vi "Timer.vi"() -> ()   [LabVIEW 2012]
uses:
  SAPI_TTS_Library_v110/SAPI TTS Library/SubVIs/SAPI_Speak_Text_String_SubVI.vi
  <vilib>/Instr/_visa.llb/VISA Configure Serial Port (Instr).vi
  SAPI_TTS_Library_v110/SAPI TTS Library/SAPI.TTS.lvlib
panel:
  in  "Boolean 2":bool
  out "Start":bool
  out "Speaking... 3":bool
  in  "Volume 3":i32(slide)=100 min=0 max=100 scale=0.0..100.0
  in  "Rate 3":i32(slide) min=-10 max=10 scale=-10.0..10.0
  in  "Output Device 3":u16(ring) items=["Speakers (Realtek High Definition Audio)"]
  in  "TTS Voice 3":u16(ring) items=["Microsoft Anna - English (United States)"]
  out "Speaking... 2":bool
  in  "Volume 2":i32(slide)=100 min=0 max=100 scale=0.0..100.0
  in  "Rate 2":i32(slide) min=-10 max=10 scale=-10.0..10.0
  in  "Output Device 2":u16(ring) items=["Speakers (Realtek High Definition Audio)"]
  in  "TTS Voice 2":u16(ring) items=["Microsoft Anna - English (United States)"]
  in  "String to Speak 2":string
  in  "Boolean":bool
  out "最高纪录 (Max Record)":dbl format="%.6f"
  in  "String to Speak":string
  in  "TTS Voice":u16(ring) items=["Microsoft Anna - English (United States)"]
  in  "Output Device":u16(ring) items=["Speakers (Realtek High Definition Audio)"]
  in  "Rate":i32(slide) min=-10 max=10 scale=-10.0..10.0
  in  "Volume":i32(slide)=100 min=0 max=100 scale=0.0..100.0
  out "Speaking...":bool
  out "已用时间 (Elasped Time)":dbl format="%.3f"
  out "LastTimeDetected":dbl
  out "单圈时间 (Lap Time)":dbl format="%.3f"
  in  "启动 / 停止":bool
  in  "赛道总长度":dbl
  in  "串口号":refnum<visa-resource-name>
  out "平均速度 (Average Speed)":dbl format="%.6f"
  # "武汉工程大学 \n”Freescale“赛道计时器"
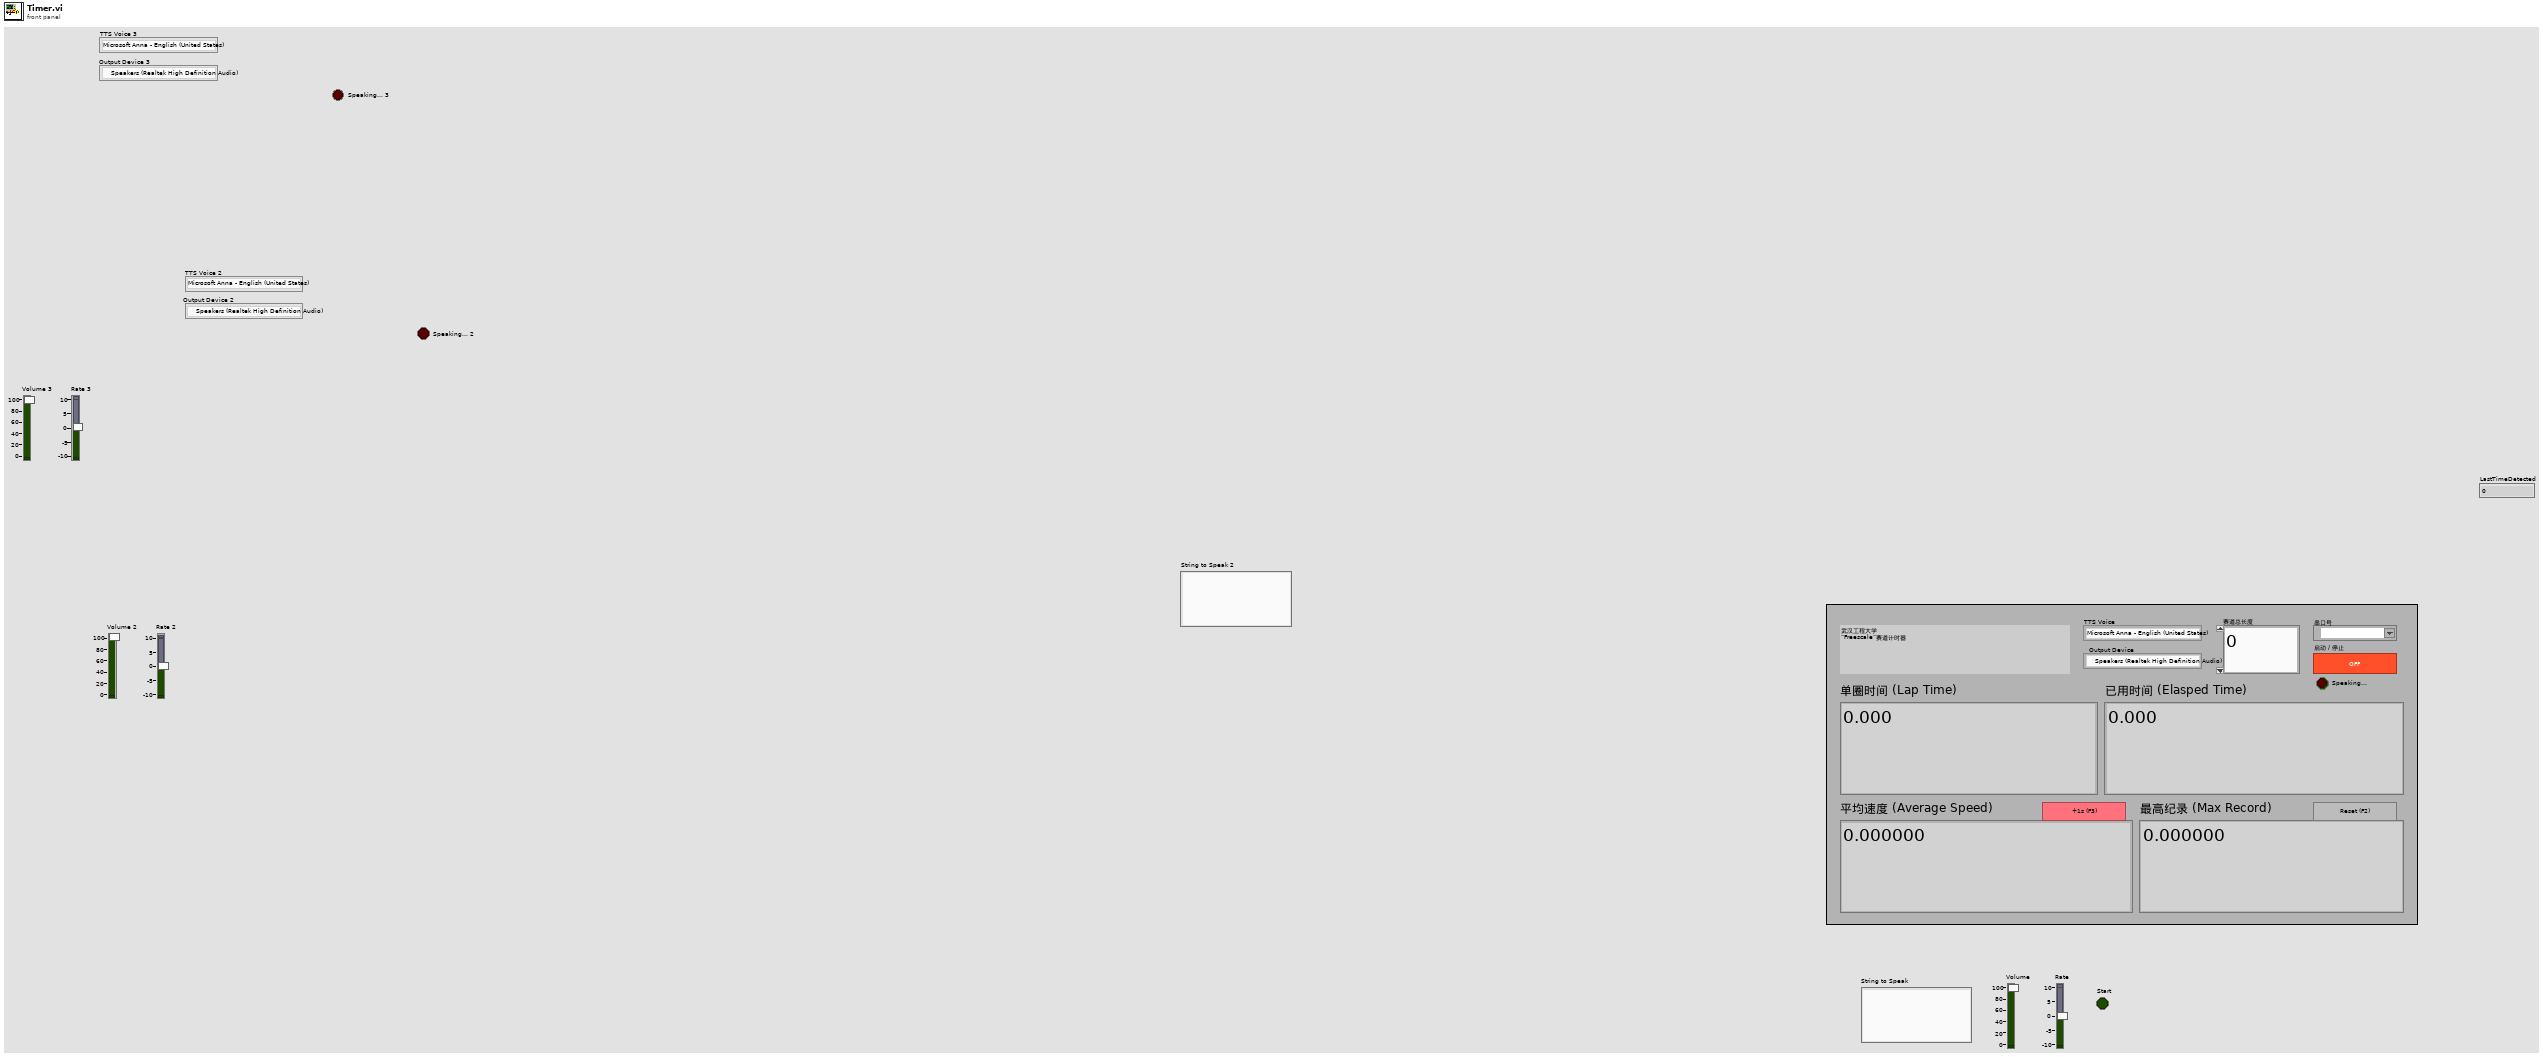
[diagram p1: front panel]
types:
  T1 = typedef "SAPI.TTS.lvlib/Speech object references.ctl" = cluster{"SpeechLib.ISpeechVoice":refnum<k7>, "GetVoices":refnum<k7>, "GetAudioOutputs":refnum<k7>}
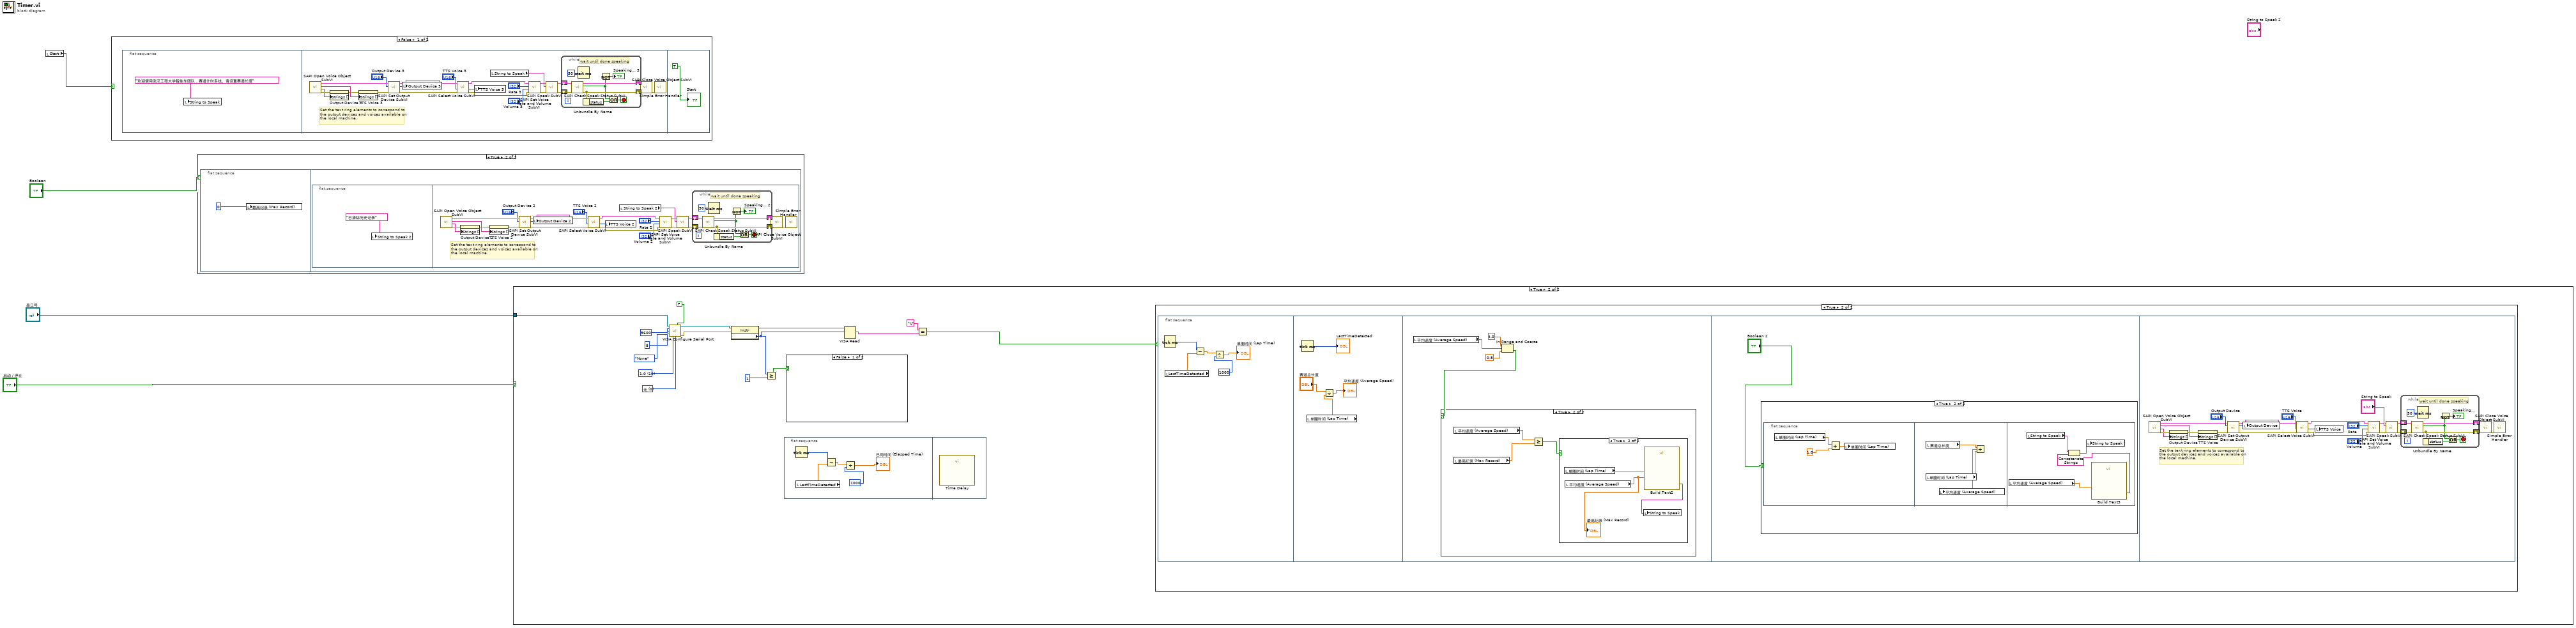
[diagram p0: block diagram]
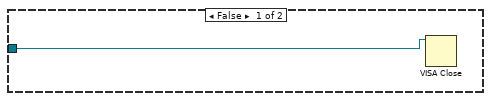
[diagram p4: hidden frame]
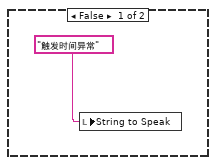
[diagram p6: hidden frame]
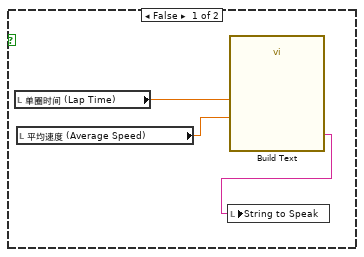
[diagram p7: hidden frame]
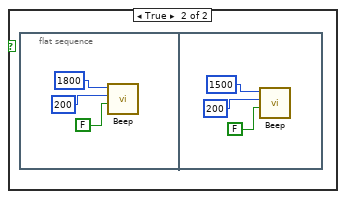
[diagram p9: hidden frame]
diagram:
  n1 = local read "Start"() -> (w1:bool)
  n2 = case shown="False" w1 {
    frame False {
      n3 = flat-sequence {
        frame #0 {
          n4 = local write "String to Speak"("欢迎使用武汉工程大学智能车团队，赛道计时系统。请设置赛道长度") -> ()
        }
        frame #1 {
          # "Set the text ring elements to correspond to\nthe output devices and voices available on\nthe local machine."
          n5 = call "SAPI Open Voice Object SubVI.vi"() -> ("error out"=w19:errorcluster, "AudioOutputs"=w20:string[], "Voice Names"=w14:string[], "speech object references"=w18:T1)  [unwired: 8 in]
          n6 = property on="Output Device 3" class="Ring (strict)"(error in=w19, "Strings []"=w20) -> (error out=w11:errorcluster)  [unwired: 1 in, 1 out]
          n7 = property on="TTS Voice 3" class="Ring (strict)"(error in=w11, "Strings []"=w14) -> (error out=w10:errorcluster)  [unwired: 1 in, 1 out]
          n8 = call "SAPI Set Output Device SubVI.vi"("error in (no error)"=w10, "Device Number"="Output Device 3", "speech object references"=w18) -> ("error out"=w9:errorcluster, "Device Number"=w15:u16, "speech object references (out)"=w17:T1)  [unwired: 6 in]
          n9 = local write "Output Device 3"(w15) -> ()
          n10 = call "SAPI Select Voice SubVI.vi"("error in (no error)"=w9, "Voice Index (default voice: 0)"="TTS Voice 3", "speech object references"=w17) -> ("error out"=w24:errorcluster, "Voice Index (coerced)"=w12:u16, "speech object references (out)"=w26:T1)  [unwired: 6 in]
          n11 = local write "TTS Voice 3"(w12) -> ()
          n12 = local read "String to Speak"() -> (w6:string)
          n13 = call "SAPI Set Voice Rate and Volume SubVI.vi"("error in (no error)"=w24, "Volume (0 to 100: 100)"="Volume 3", "Speech Rate (-10 to 10: 0)"="Rate 3", "speech object references"=w26) -> ("error out"=w23:errorcluster, "speech object references (out)"=w25:T1)  [unwired: 6 in]
          n14 = call-poly "SAPI Speak SubVI.vi"("error in (no error)"=w23, "Text to speak"=w6, "speech object references"=w25) -> ("error out"=w28:errorcluster, "speech object references (out)"=w29:T1)  [unwired: 7 in]
          n15 = while {
            shift-right: [w33] -> w7
            shift-left: w28 -> [w37]
            shift-right: [w34] -> w8
            shift-left: w29 -> [w38]
            stop <- w35 stop-if-true
            # "wait until done speaking"
            n16 = call "SAPI Check Speak Status SubVI.vi"("error in (no error)"=w37, "speech object references"=w38) -> ("error out"=w33:errorcluster, "Status (T: Done)"=w32:bool, "speech object references (out)"=w34:T1)  [unwired: 7 in]
            n17 = Wait (ms)(milliseconds to wait=u32 50) -> ()  [unwired: 1 out]
            n18 = Unbundle By Name(w33) -> ("status"=w36:bool)
            n19 = Not(x=w32) -> (.not. x?=→"Speaking... 3":bool)
            n20 = Or(x=w32, y=w36) -> (x .or. y?=w35:bool)
          }
          n21 = call "SAPI Close Voice Object SubVI.vi"("error in (no error)"=w7, "speech object references"=w8) -> ("error out"=w27:errorcluster)  [unwired: 9 in]
          n22 = call <vilib>:"Simple Error Handler.vi"("error in (no error)"=w27) -> ()  [unwired: 4 in, 5 out]
        }
        frame #2 {
          "Start" <- TRUE
        }
      }
    }
    frame True {
    }
  }
  n23 = case shown="True" "Boolean" {
    frame False {
    }
    frame True {
      n24 = flat-sequence {
        frame #0 {
          n25 = local write "最高纪录 (Max Record)"(0) -> ()
        }
        frame #1 {
          n26 = flat-sequence {
            frame #0 {
              n27 = local write "String to Speak 2"("已清除历史记录") -> ()
            }
            frame #1 {
              # "Set the text ring elements to correspond to\nthe output devices and voices available on\nthe local machine."
              n28 = call "SAPI Open Voice Object SubVI.vi"() -> ("error out"=w55:errorcluster, "AudioOutputs"=w56:string[], "Voice Names"=w50:string[], "speech object references"=w54:T1)  [unwired: 8 in]
              n29 = property on="Output Device 2" class="Ring (strict)"(error in=w55, "Strings []"=w56) -> (error out=w47:errorcluster)  [unwired: 1 in, 1 out]
              n30 = property on="TTS Voice 2" class="Ring (strict)"(error in=w47, "Strings []"=w50) -> (error out=w46:errorcluster)  [unwired: 1 in, 1 out]
              n31 = call "SAPI Set Output Device SubVI.vi"("error in (no error)"=w46, "Device Number"="Output Device 2", "speech object references"=w54) -> ("error out"=w45:errorcluster, "Device Number"=w51:u16, "speech object references (out)"=w53:T1)  [unwired: 6 in]
              n32 = local write "Output Device 2"(w51) -> ()
              n33 = call "SAPI Select Voice SubVI.vi"("error in (no error)"=w45, "Voice Index (default voice: 0)"="TTS Voice 2", "speech object references"=w53) -> ("error out"=w60:errorcluster, "Voice Index (coerced)"=w48:u16, "speech object references (out)"=w62:T1)  [unwired: 6 in]
              n34 = local write "TTS Voice 2"(w48) -> ()
              n35 = local read "String to Speak 2"() -> (w42:string)
              n36 = call "SAPI Set Voice Rate and Volume SubVI.vi"("error in (no error)"=w60, "Volume (0 to 100: 100)"="Volume 2", "Speech Rate (-10 to 10: 0)"="Rate 2", "speech object references"=w62) -> ("error out"=w59:errorcluster, "speech object references (out)"=w61:T1)  [unwired: 6 in]
              n37 = call-poly "SAPI Speak SubVI.vi"("error in (no error)"=w59, "Text to speak"=w42, "speech object references"=w61) -> ("error out"=w64:errorcluster, "speech object references (out)"=w65:T1)  [unwired: 7 in]
              n38 = while {
                shift-right: [w69] -> w43
                shift-left: w64 -> [w73]
                shift-right: [w70] -> w44
                shift-left: w65 -> [w74]
                stop <- w71 stop-if-true
                # "wait until done speaking"
                n39 = call "SAPI Check Speak Status SubVI.vi"("error in (no error)"=w73, "speech object references"=w74) -> ("error out"=w69:errorcluster, "Status (T: Done)"=w68:bool, "speech object references (out)"=w70:T1)  [unwired: 7 in]
                n40 = Wait (ms)(milliseconds to wait=u32 50) -> ()  [unwired: 1 out]
                n41 = Unbundle By Name(w69) -> ("status"=w72:bool)
                n42 = Not(x=w68) -> (.not. x?=→"Speaking... 2":bool)
                n43 = Or(x=w68, y=w72) -> (x .or. y?=w71:bool)
              }
              n44 = call "SAPI Close Voice Object SubVI.vi"("error in (no error)"=w43, "speech object references"=w44) -> ("error out"=w63:errorcluster)  [unwired: 9 in]
              n45 = call <vilib>:"Simple Error Handler.vi"("error in (no error)"=w63) -> ()  [unwired: 4 in, 5 out]
            }
          }
        }
      }
    }
  }
  n46 = case shown="True" "启动 / 停止" {
    tunnel: "串口号" -> [w75 w91]
    frame False {
      n47 = VISA Close(VISA resource name=w75) -> ()  [unwired: 1 in, 1 out]
    }
    frame True {
      w85 = u16 0 items=["无", "XON/XOFF", "RTS/CTS", "XON/XOFF & RTS/CTS", "DTR/DSR", "XON/XOFF & DTR/DSR"] ("flow control (0:none)")
      w86 = u16 10 items=["1.0"=10, "1.5"=15, "2.0"=20] ("stop bits (10: 1 bit)")
      n48 = call-poly "VISA Configure Serial Port"("VISA resource name"=w91, "Enable Termination\nChar (T)"=FALSE ("Enable Termination\nChar (T)"), "baud rate (9600)"=u32 9600, "data bits (8)"=u16 8, "parity (0:none)"=enum16{"None", "Odd", "Even", "Mark", "Space"}."None", "stop bits (10: 1 bit)"=w86, "flow control (0:none)"=w85) -> ("VISA resource name out"=w84:refnum<visa-resource-name>, "error out"=w83:errorcluster)  [unwired: 7 in]
      n49 = property class="Instr"(reference=w84, error in=w83) -> (reference out=w82:refnum<visa-resource-name>, "Serial Settings:Number of Bytes at Serial Port"=w81:u32)  [unwired: 1 out]
      n50 = Greater Or Equal?(x=w81, y=u32 1) -> (x >= y?=w79:bool)
      n51 = flat-sequence {
        frame #0 {
          n52 = Tick Count (ms)() -> (millisecond timer value=w94:u32)
          n53 = local read "LastTimeDetected"() -> (w95:dbl)
          n54 = Subtract(x=w94, y=w95) -> (x-y=w93:dbl)
          n55 = Divide(x=w93, y=1000) -> (x/y=→"已用时间 (Elasped Time)":dbl)
        }
        frame #1 {
          n56 = call "Time Delay"() -> ()  [unwired: 11 in, 1 out]
        }
      }
      n57 = case shown="False" w79 {
        frame False {
        }
        frame True {
          n58 = flat-sequence {
            frame #0 {
              n59 = call <vilib>:"Beep.vi"("use system alert? (T)"=FALSE ("Enable Termination\nChar (T)"), "duration (msec)"=200, "frequency (Hz)"=1800) -> ()  [unwired: 9 in]
            }
            frame #1 {
              n60 = call <vilib>:"Beep.vi"("use system alert? (T)"=FALSE ("Enable Termination\nChar (T)"), "duration (msec)"=200, "frequency (Hz)"=1500) -> ()  [unwired: 9 in]
            }
          }
        }
      }
      n61 = VISA Read(VISA resource name=w82, byte count=w81) -> (read buffer=w78:string)  [unwired: 1 in, 3 out]
      n62 = Equal?(x="U", y=w78) -> (x = y?=w76:bool)
      n63 = case shown="True" w76 {
        frame False {
        }
        frame True {
          n64 = flat-sequence {
            frame #0 {
              n65 = Tick Count (ms)() -> (millisecond timer value=w100:u32)
              n66 = local read "LastTimeDetected"() -> (w101:dbl)
              n67 = Subtract(x=w100, y=w101) -> (x-y=w99:dbl)
              n68 = Divide(x=w99, y=1000) -> (x/y=→"单圈时间 (Lap Time)":dbl)
            }
            frame #1 {
              n69 = Tick Count (ms)() -> (millisecond timer value=→"LastTimeDetected":u32)
              n70 = local read "单圈时间 (Lap Time)"() -> (w103:dbl)
              n71 = Divide(x="赛道总长度", y=w103) -> (x/y=→"平均速度 (Average Speed)":dbl)
            }
            frame #2 {
              n72 = local read "平均速度 (Average Speed)"() -> (w109:dbl)
              n73 = In Range and Coerce(upper limit=4.0, x=w109, lower limit=0.5) -> (In Range?=w106:bool)  [unwired: 1 out]
              n74 = case shown="True" w106 {
                frame False {
                  n75 = local write "String to Speak"("触发时间异常") -> ()
                }
                frame True {
                  n76 = local read "平均速度 (Average Speed)"() -> (w113:dbl)
                  n77 = local read "最高纪录 (Max Record)"() -> (w112:dbl)
                  n78 = Greater Or Equal?(x=w113, y=w112) -> (x >= y?=w111:bool)
                  n79 = case shown="True" w111 {
                    frame False {
                      n80 = local read "单圈时间 (Lap Time)"() -> (w114:dbl)
                      n81 = local read "平均速度 (Average Speed)"() -> (w115:dbl)
                      n82 = call "Build Text"("time"=w114, "speed"=w115) -> ("Result"=w116:string)  [unwired: 12 in, 1 out]
                      n83 = local write "String to Speak"(w116) -> ()
                    }
                    frame True {
                      n84 = local read "单圈时间 (Lap Time)"() -> (w118:dbl)
                      n85 = local read "平均速度 (Average Speed)"() -> (w117:dbl)
                      "最高纪录 (Max Record)" <- w117
                      n86 = call "Build Text2"("time"=w118, "speed"=w117) -> ("Result"=w119:string)  [unwired: 12 in, 1 out]
                      n87 = local write "String to Speak"(w119) -> ()
                    }
                  }
                }
              }
            }
            frame #3 {
              n88 = case shown="True" "Boolean 2" {
                frame False {
                }
                frame True {
                  n89 = flat-sequence {
                    frame #0 {
                      n90 = local read "单圈时间 (Lap Time)"() -> (w123:dbl)
                      n91 = Add(x=w123, y=1.0) -> (x+y=w121:dbl)
                      n92 = local write "单圈时间 (Lap Time)"(w121) -> ()
                    }
                    frame #1 {
                      n93 = local read "单圈时间 (Lap Time)"() -> (w125:dbl)
                      n94 = local read "赛道总长度"() -> (w126:dbl)
                      n95 = Divide(x=w126, y=w125) -> (x/y=w124:dbl)
                      n96 = local write "平均速度 (Average Speed)"(w124) -> ()
                    }
                    frame #2 {
                      n97 = local read "平均速度 (Average Speed)"() -> (w128:dbl)
                      n98 = local read "String to Speak"() -> (w130:string)
                      n99 = call "Build Text3"("speed"=w128) -> ("Result"=w127:string)  [unwired: 13 in, 1 out]
                      n100 = Concatenate Strings(w130, w127) -> (w129:string)
                      n101 = local write "String to Speak"(w129) -> ()
                    }
                  }
                }
              }
            }
            frame #4 {
              # "Set the text ring elements to correspond to\nthe output devices and voices available on\nthe local machine."
              n102 = call "SAPI Open Voice Object SubVI.vi"() -> ("error out"=w141:errorcluster, "AudioOutputs"=w140:string[], "Voice Names"=w146:string[], "speech object references"=w142:T1)  [unwired: 8 in]
              n103 = property on="Output Device" class="Ring (strict)"(error in=w141, "Strings []"=w140) -> (error out=w149:errorcluster)  [unwired: 1 in, 1 out]
              n104 = property on="TTS Voice" class="Ring (strict)"(error in=w149, "Strings []"=w146) -> (error out=w150:errorcluster)  [unwired: 1 in, 1 out]
              n105 = call "SAPI Set Output Device SubVI.vi"("error in (no error)"=w150, "Device Number"="Output Device", "speech object references"=w142) -> ("error out"=w151:errorcluster, "Device Number"=w145:u16, "speech object references (out)"=w143:T1)  [unwired: 6 in]
              n106 = local write "Output Device"(w145) -> ()
              n107 = call "SAPI Select Voice SubVI.vi"("error in (no error)"=w151, "Voice Index (default voice: 0)"="TTS Voice", "speech object references"=w143) -> ("error out"=w136:errorcluster, "Voice Index (coerced)"=w148:u16, "speech object references (out)"=w134:T1)  [unwired: 6 in]
              n108 = local write "TTS Voice"(w148) -> ()
              n109 = call "SAPI Set Voice Rate and Volume SubVI.vi"("error in (no error)"=w136, "Volume (0 to 100: 100)"="Volume", "Speech Rate (-10 to 10: 0)"="Rate", "speech object references"=w134) -> ("error out"=w137:errorcluster, "speech object references (out)"=w135:T1)  [unwired: 6 in]
              n110 = call-poly "SAPI Speak SubVI.vi"("error in (no error)"=w137, "Text to speak"="String to Speak", "speech object references"=w135) -> ("error out"=w132:errorcluster, "speech object references (out)"=w131:T1)  [unwired: 7 in]
              n111 = while {
                shift-right: [w158] -> w153
                shift-left: w132 -> [w162]
                shift-right: [w159] -> w152
                shift-left: w131 -> [w163]
                stop <- w160 stop-if-true
                # "wait until done speaking"
                n112 = call "SAPI Check Speak Status SubVI.vi"("error in (no error)"=w162, "speech object references"=w163) -> ("error out"=w158:errorcluster, "Status (T: Done)"=w157:bool, "speech object references (out)"=w159:T1)  [unwired: 7 in]
                n113 = Wait (ms)(milliseconds to wait=u32 50) -> ()  [unwired: 1 out]
                n114 = Unbundle By Name(w158) -> ("status"=w161:bool)
                n115 = Not(x=w157) -> (.not. x?=→"Speaking...":bool)
                n116 = Or(x=w157, y=w161) -> (x .or. y?=w160:bool)
              }
              n117 = call "SAPI Close Voice Object SubVI.vi"("error in (no error)"=w153, "speech object references"=w152) -> ("error out"=w133:errorcluster)  [unwired: 9 in]
              n118 = call <vilib>:"Simple Error Handler.vi"("error in (no error)"=w133) -> ()  [unwired: 4 in, 5 out]
            }
          }
        }
      }
    }
  }
